vi "Initialize PID Settings.vi"(8 "error in (no error)":errorcluster, 10 "PID Settings":refnum<vi>, 11 "Item Ref in":T1 format="%.0x") -> (0 "error out":errorcluster, 3 "Item Ref out":T1=18446744073709551615 format="%.0x")   [LabVIEW 2019, in "Control Addon System Explorer.lvlib"]
uses:
  Control Addon System Explorer.lvlib
  <vilib>/NI VeriStand/Custom Device API/Custom Device Item Ref.ctl
  Types/Action.ctl
  Addon Shared/SubVIs/Constants.vi
  <vilib>/NI VeriStand/Custom Device API/NI VeriStand - Get Item Property.vi
  <vilib>/NI VeriStand/Custom Device API/Get Item Property (Boolean).vi
  <vilib>/NI VeriStand/Custom Device API/Get Item Property (String).vi
  <vilib>/NI VeriStand/Custom Device API/NI VeriStand - Set Item Property.vi
  <vilib>/NI VeriStand/Custom Device API/Set Item Property (Boolean).vi
  <vilib>/NI VeriStand/Custom Device API/Set Item Property (String).vi
  <vilib>/NI VeriStand/Custom Device API/Custom Device API.lvlib
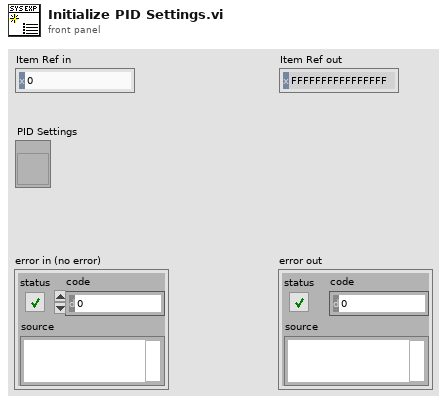
[diagram p1: front panel]
types:
  T1 = typedef "Custom Device API.lvlib/Custom Device Item Ref.ctl" = u64
  T2 = typedef "Control Addon System Explorer.lvlib/Action.ctl" = enum16{"Get", "Set"}
  T3 = typedef "Control Addon Shared.lvlib/PID Parameters.ctl" = cluster{"Enable Live Updates":bool, "Enable Gain Scheduling":bool, "PID Parameters":dbl[][]}
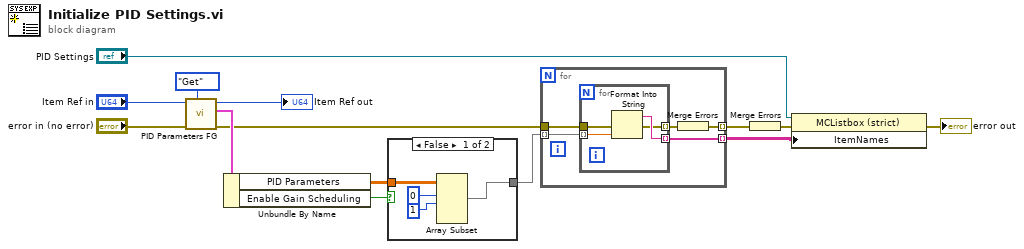
[diagram p0: block diagram]
diagram:
  n1 = call "PID Parameters FG.vi"("Action"=Action."Get", "error in (no error)"="error in (no error)", "Node Ptr"="Item Ref in") -> ("error out"=w8:errorcluster, "Parameters"=w10:T3, "Item Ref out"=→"Item Ref out":T1)  [unwired: 6 in]
  n2 = Unbundle By Name(w10) -> ("PID Parameters"=w2:dbl[][], "Enable Gain Scheduling"=w3:bool)
  n3 = case shown="False" w3 {
    tunnel: w2 -> [w18 w19]
    tunnel: [w15 w19] -> w1
    frame False {
      n4 = Array Subset(array=w18, index (row)=0 ("index"), length (row)=1 ("length")) -> (w15:dbl[][])  [unwired: 2 in]
    }
    frame True {
    }
  }
  n5 = for {
    tunnel: w1 -> [w24] mode=indexing
    tunnel: [w23] -> w6 mode=indexing
    tunnel: [w22] -> w13 mode=indexing
    tunnel: w8 -> [w20]
    n6 = for {
      tunnel: w24 -> [w25] mode=indexing
      tunnel: [w28] -> w23 mode=indexing
      tunnel: [w27] -> w21 mode=indexing
      tunnel: w20 -> [w26]
      n7 = Format Into String(error in=w26, w25) -> (resulting string=w28:string, error out=w27:errorcluster)  [unwired: 2 in]
    }
    n8 = Merge Errors(w21) -> (w22:errorcluster)
  }
  n9 = Merge Errors(w13) -> (w7:errorcluster)
  n10 = property class="MCListbox (strict)"(reference="PID Settings", error in=w7, "ItemNames"=w6) -> (error out=→"error out":errorcluster)  [unwired: 1 out]
